vi "Disgusting array concatenation.vi"(4 "Trigger":bool, 6 "COUNTIN":u32, 9 "LongitudeArray":dbl[](array[numeric]), 10 "LatitudeArray":dbl[](array[numeric])) -> (0 "CurrentLon":dbl, 1 "CurrentLat":dbl, 2 "PastLon":dbl, 3 "PastLat":dbl, 5 "COUNTOUT":u32)   [LabVIEW 2017]
panel:
  # "This VI places the current GPS data in an array and then seperates it and the previous GPS data from that array for decision making down the road.\nIt only triggers fully whenver the count reaches the desired amount indicating that its time to reevaluate where the robot is at, where it needs to go and how it will get there."
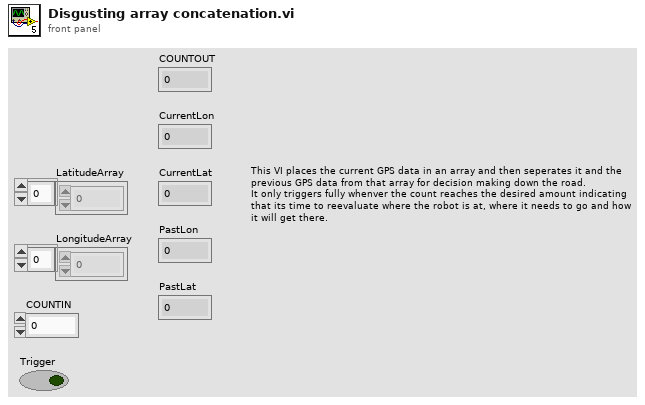
[diagram p1: front panel]
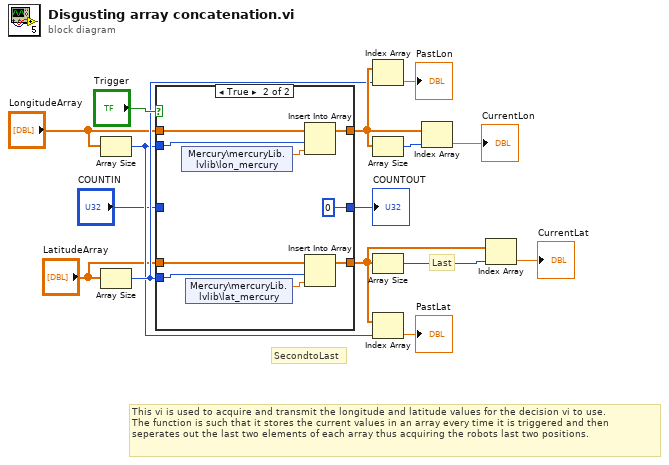
[diagram p0: block diagram]
diagram:
  # "This vi is used to acquire and transmit the longitude and latitude values for the decision vi to use.\nThe function is such that it stores the current values in an array every time it is triggered and then seperates out the last two elements of each array thus acquiring the robots last two positions."
  # "Last"
  # "SecondtoLast"
  n1 = Array Size(array="LongitudeArray") -> (size(s)=w5:i32)
  n2 = Array Size(array="LatitudeArray") -> (size(s)=w6:i32)
  n3 = case shown="True" "Trigger" {
    tunnel: "COUNTIN" -> [w18 _]
    tunnel: [w18 0] -> w2
    tunnel: "LatitudeArray" -> [w17 w22]
    tunnel: "LongitudeArray" -> [w16 w26]
    tunnel: [w17 w25] -> w8
    tunnel: [w16 w24] -> w10
    tunnel: w6 -> [_ w23]
    tunnel: w5 -> [_ w21]
    frame False {
    }
    frame True {
      n4 = shared-variable "Mercury\\mercuryLib.lvlib\\lon_mercury"() -> (w19:dbl)  [unwired: 1 in, 1 out]
      n5 = shared-variable "Mercury\\mercuryLib.lvlib\\lat_mercury"() -> (w20:dbl)  [unwired: 1 in, 1 out]
      n6 = Insert Into Array(array=w26, index=w21, new element=w19) -> (w24:dbl[])
      n7 = Insert Into Array(array=w22, index=w23, new element=w20) -> (w25:dbl[])
    }
  }
  "COUNTOUT" <- w2
  n8 = Index Array(array=w10, index=w6) -> (element=→"PastLon":dbl)
  n9 = Array Size(array=w10) -> (size(s)=w9:i32)
  n10 = Array Size(array=w8) -> (size(s)=w7:i32)
  n11 = Index Array(array=w8, index=w5) -> (element=→"PastLat":dbl)
  n12 = Index Array(array=w10, index=w9) -> (element=→"CurrentLon":dbl)
  n13 = Index Array(array=w8, index=w7) -> (element=→"CurrentLat":dbl)
